vi "XYZ2MoveCommand.vi"(9 "Z":dbl, 10 "Y":dbl, 11 "X":dbl) -> (3 "String":string)   [LabVIEW 2016]
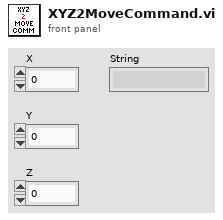
[diagram p1: front panel]
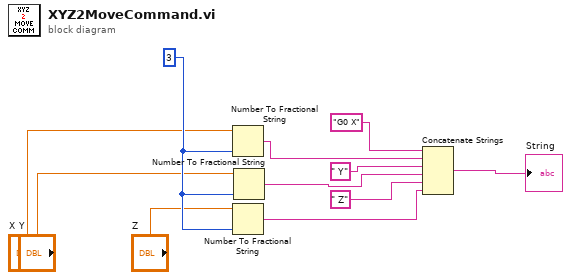
[diagram p0: block diagram]
diagram:
  w4 = 3
  n1 = Number To Fractional String(number="X", precision (6)=w4) -> (F-format string=w5:string)  [unwired: 2 in]
  n2 = Number To Fractional String(number="Z", precision (6)=w4) -> (F-format string=w10:string)  [unwired: 2 in]
  n3 = Number To Fractional String(number="Y", precision (6)=w4) -> (F-format string=w8:string)  [unwired: 2 in]
  n4 = Concatenate Strings("G0 X", w5, " Y", w8, " Z", w10) -> (→"String":string)
